vi "AM_Write_Freq.vi"(3 "error in (no error)":errorcluster, 4 "Delay / ms":u32, 5 "f / Hz":dbl min=0.0 max=3.3, 6 "VISA resource name":refnum<visa-resource-name>) -> (0 "error out":errorcluster, 1 "Cmd":string, 2 "VISA resource name 2":refnum<visa-resource-name>)   [LabVIEW 2018]
doc: "Send a command to the Arduino Micro telling it to change SparkFun MiniGen Frequencys\nInput frequency must be in the range 100 Hz <= f <= 3 MHz\n\nR. Sheehan 13 - 11 - 2020"
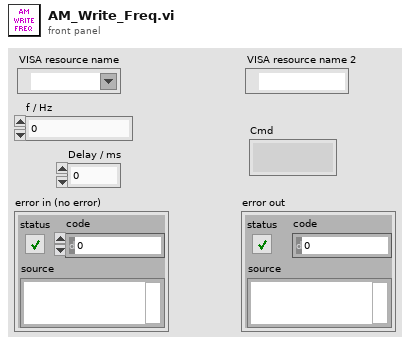
[diagram p1: front panel]
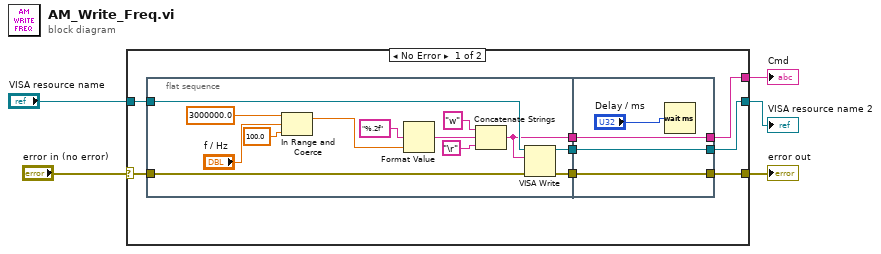
[diagram p0: block diagram]
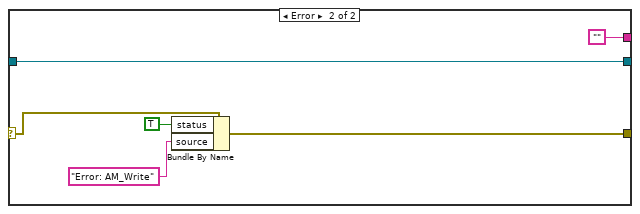
[diagram p2: hidden frame]
diagram:
  n1 = case shown="No Error" "error in (no error)" {
    selector: "error in (no error)" -> [w12 w36]
    tunnel: [w9 w35] -> w4
    tunnel: "VISA resource name" -> [w13 w32]
    tunnel: [w10 w32] -> w2
    tunnel: [w11 ""] -> w1
    frame No Error {
      n2 = flat-sequence {
        tunnel: w13 -> [w22]
        tunnel: w12 -> [w21]
        tunnel: [w20] -> w8
        tunnel: [w19] -> w7
        tunnel: [w18] -> w6
        tunnel: [w28] -> w9
        tunnel: [w29] -> w10
        tunnel: [w30] -> w11
        tunnel: w8 -> [w30]
        tunnel: w7 -> [w29]
        tunnel: w6 -> [w28]
        frame #0 {
          n3 = In Range and Coerce(upper limit=3000000.0, x="f / Hz", lower limit=100.0) -> (coerced(x)=w14:dbl)  [unwired: 1 out]
          n4 = Format Value(format string="%.2f", value (0)=w14) -> (output string=w23:string)  [unwired: 1 in]
          n5 = Concatenate Strings("w" ("string"), w23, "\r") -> (w20:string)
          n6 = VISA Write(VISA resource name=w22, write buffer=w20, error in (no error)=w21) -> (VISA resource name out=w19:refnum<visa-resource-name>, error out=w18:errorcluster)  [unwired: 1 out]
        }
        frame #1 {
          n7 = Wait (ms)(milliseconds to wait="Delay / ms") -> ()  [unwired: 1 out]
        }
      }
    }
    frame Error {
      n8 = Bundle By Name(cluster=w36, "status"=TRUE, "source"="Error: AM_Write") -> (w35:errorcluster)
    }
  }
  "error out" <- w4
  "VISA resource name 2" <- w2
  "Cmd" <- w1
